vi "AMZ_S3_APIHLP_Generate Event XML.vi"(11 "Events":T1[](array[typedef])) -> (3 "Event XML":string)   [LabVIEW 2015, in "LV Interface for Amazon S3.lvlib"]
uses:
  LV Interface for Amazon S3.lvlib
  Typedefs/AMZ_S3_Event.ctl
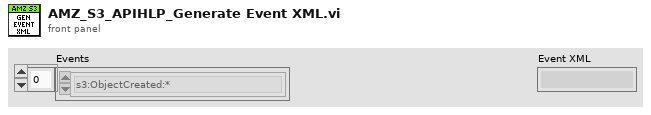
[diagram p1: front panel]
types:
  T1 = typedef "LV Interface for Amazon S3.lvlib/AMZ_S3_Event.ctl" = enum16{"s3:ObjectCreated:*", "s3:ObjectCreated:Put", "s3:ObjectCreated:Post", "s3:ObjectCreated:Copy", "s3:ObjectCreated:CompleteMultipartUpload", "s3:ObjectRemoved:*", "s3:ObjectRemoved:Delete", "s3:ObjectRemoved:DeleteMarkerCreated", "s3:ReducedRedundancyLostObject"}
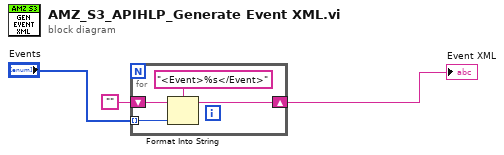
[diagram p0: block diagram]
diagram:
  n1 = for {
    tunnel: "Events" -> [w5] mode=indexing
    shift-right: [w6] -> w3
    shift-left: "" -> [w7]
    n2 = Format Into String(format string="<Event>%s</Event>", initial string=w7, w5) -> (resulting string=w6:string)  [unwired: 1 in, 1 out]
  }
  "Event XML" <- w3
